vi "test Correct Acyclic Labels In Log.vi"(8 "error in":errorcluster, 11 "TestCase in":refnum<class "Logging Loopback.lvclass">) -> (0 "error out":errorcluster, 3 "TestCase out":refnum<class "Logging Loopback.lvclass">)   [LabVIEW 2020, in "Logging Loopback.lvclass"]
uses:
  Logging Loopback.lvclass
  C:/Users/nitest/Desktop/Git 2020/niveristand-custom-device-testing-tools/VeriStandTestCase/VeriStandTestCase.lvclass
  Logging Loopback.lvclass/Logging Loopback.ctl
  4890de3c-2bf7-434e-869c-ee5afaf04248.vi
  <vilib>/NI VeriStand/Execution/Workspace/NI VeriStand - Set Multiple Channel Values.vi
  <vilib>/WebDAVClient/Advanced/Get Buffer.vi
  <vilib>/addons/_JKI Toolkits/VI Tester/TestCase.llb/TestCase.lvclass
  <vilib>/WebDAVClient/NI_WebDAV.lvlib
  <vilib>/NI VeriStand/Execution/Workspace/NI_VS Workspace ExecutionAPI.lvlib
  C:/Program Files (x86)/National Instruments/LabVIEW 2020/vi.lib/addons/_JKI Toolkits/VI Tester/TestCase.llb/TestCase.lvclass
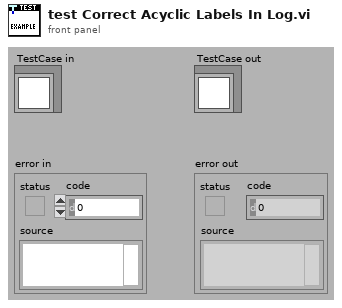
[diagram p1: front panel]
types:
  T1 = typedef "NI_WebDAV.lvlib/SessionHandle.ctl" = refnum<k1>
  T2 = typedef "NI_VS Workspace ExecutionAPI.lvlib/WorkspaceAPI.ctl" = refnum<k24>
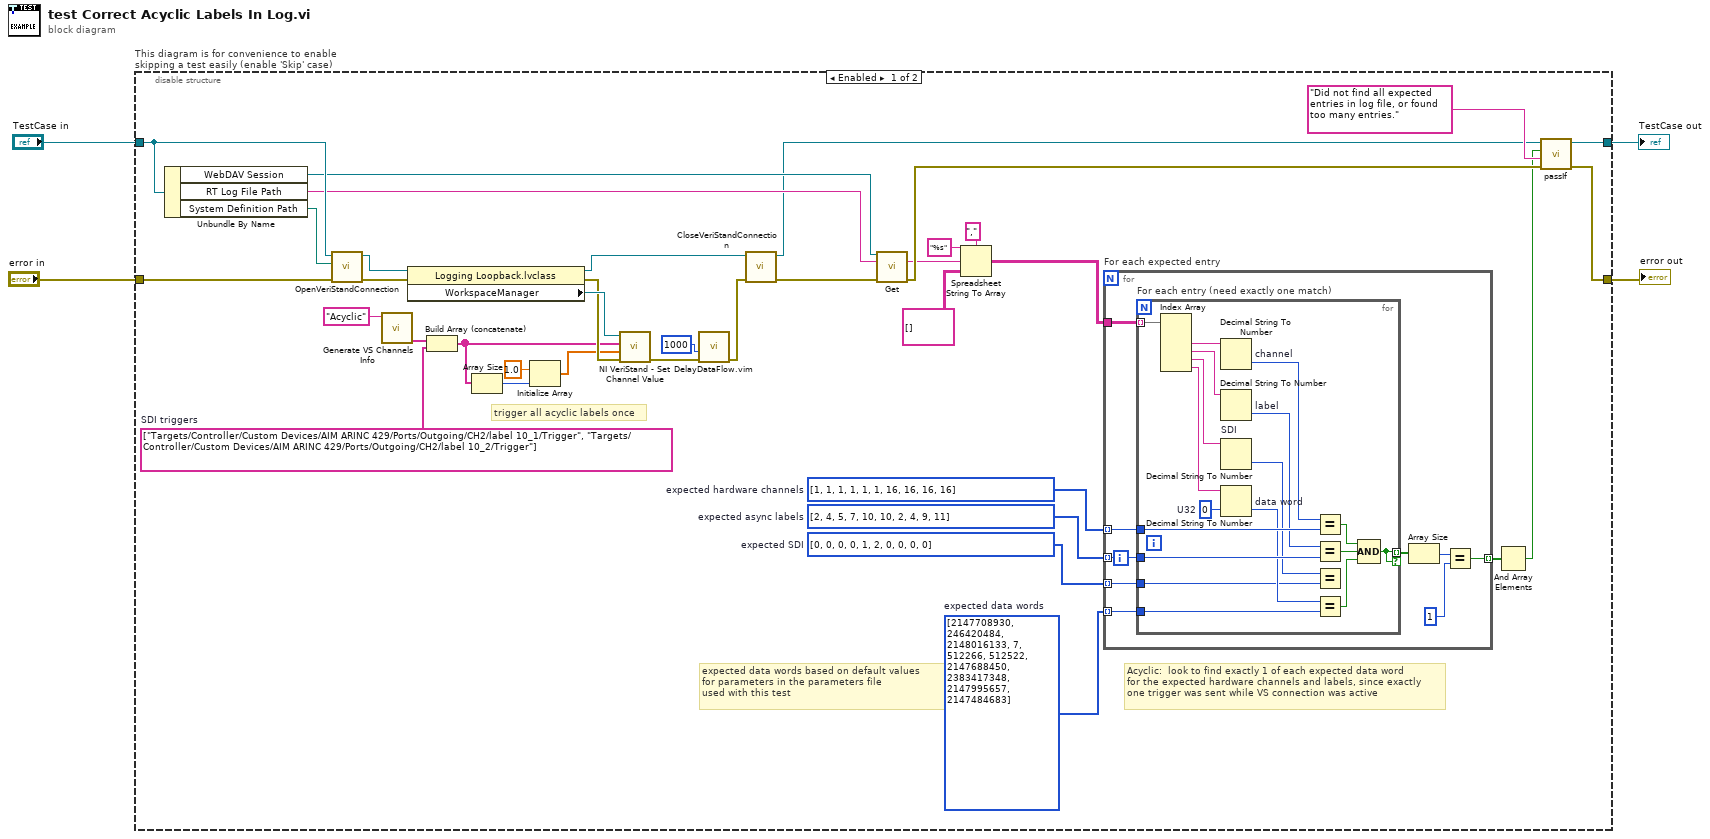
[diagram p0: block diagram]
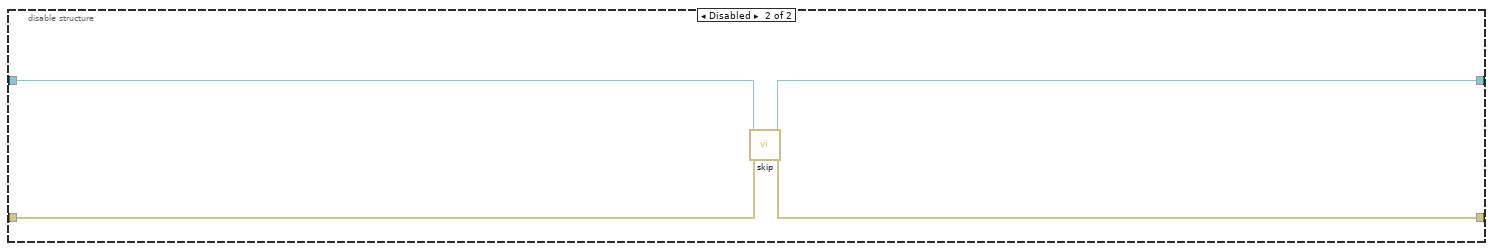
[diagram p2: hidden frame]
diagram:
  n1 = disable-structure "This diagram is for convenience to enable skipping a test easily (enable 'Skip' case)" shown="Enabled" {
    disable-tunnel: "TestCase in" -> [w39 w72]
    disable-tunnel: [w29 w70] -> w1
    disable-tunnel: [w30 w71] -> w3
    disable-tunnel: "error in" -> [w41 w69]
    frame Enabled {
      w6 = string[] ["Targets/Controller/Custom Devices/AIM ARINC 429/Ports/Outgoing/CH2/label 10_1/Trigger", "Targets/Controller/Custom Devices/AIM ARINC 429/Ports/Outgoing/CH2/label 10_2/Trigger"]  # SDI triggers
      w8 = i32[] [0, 0, 0, 0, 1, 2, 0, 0, 0, 0]  # expected SDI
      w23 = u32[] [2147708930, 246420484, 2148016133, 7, 512266, 512522, 2147688450, 2383417348, 2147995657, 2147484683]  # expected data words
      w25 = i32[] [1, 1, 1, 1, 1, 1, 16, 16, 16, 16]  # expected hardware channels
      w24 = i32[] [2, 4, 5, 7, 10, 10, 2, 4, 9, 11]  # expected async labels
      # "Acyclic:  look to find exactly 1 of each expected data word\nfor the expected hardware channels and labels, since exactly\none trigger was sent while VS connection was active"
      # "expected data words based on default values\nfor parameters in the parameters file\nused with this test"
      # "trigger all acyclic labels once"
      n2 = Unbundle By Name(w39) -> ("WebDAV Session"=w36:T1, "RT Log File Path"=w35:string, "System Definition Path"=w40:path)
      n3 = call-dynamic "OpenVeriStandConnection.vi"("error in (no error)"=w41, "System Definition File"=w40, "VeriStand Test Case in"=w39) -> ("error out"=w19:errorcluster, "VeriStand Test Case out"=w20:refnum<class "Logging Loopback.lvclass">)  [unwired: 6 in, 1 out]
      n4 = call "Generate VS Channels Info.vi"("Transfer Type"="Acyclic") -> ("Tx Trigger Channels Array"=w7:string[])  [unwired: 6 in, 4 out]
      n5 = property class="Logging Loopback.lvclass"(reference=w20, error in=w19) -> (reference out=w16:refnum<class "Logging Loopback.lvclass">, error out=w17:errorcluster, "WorkspaceManager"=w18:T2)
      n6 = Build Array (concatenate)(w7, w6) -> (w5:string[])
      n7 = Array Size(array=w5) -> (size(s)=w10:i32)
      n8 = Initialize Array(1.0, w10) -> (w12:dbl[])
      n9 = call-poly <vilib>:"NI VeriStand - Set Channel Value.vi"("error in (no error)"=w17, "Values"=w12, "Channels"=w5, "WorkspaceManager in"=w18) -> ("error out"=w14:errorcluster)  [unwired: 6 in, 1 out]
      n10 = call "DelayDataFlow.vim"("value in"=w14, "milliseconds to wait"=u32 1000) -> ("value out"=w13:errorcluster)  [unwired: 2 in, 1 out]
      n11 = call-dynamic "CloseVeriStandConnection.vi"("error in (no error)"=w13, "VeriStand Test Case in"=w16) -> ("error out"=w38:errorcluster, "VeriStand Test Case out"=w27:refnum<class "Logging Loopback.lvclass">)  [unwired: 8 in]
      n12 = call-poly <vilib>:"Get.vi"("session handle"=w36, "relative uri"=w35, "error in (no error)"=w38) -> ("data"=w34:string, "error out"=w37:errorcluster)  [unwired: 10 in, 1 out]
      n13 = Spreadsheet String To Array(delimiter (Tab)=",", format string="%s", spreadsheet string=w34, array type (2D Dbl)=string[][] []) -> (array=w26:string[][])
      n14 = for "For each expected entry" {
        tunnel: w25 -> [w49] mode=indexing
        tunnel: w24 -> [w48] mode=indexing
        tunnel: w23 -> [w47] mode=indexing
        tunnel: w26 -> [w50]
        tunnel: [w44] -> w22 mode=indexing
        tunnel: w8 -> [w42] mode=indexing
        n15 = for "For each entry (need exactly one match)" {
          tunnel: w50 -> [w68] mode=indexing
          tunnel: w49 -> [w63]
          tunnel: w48 -> [w64]
          tunnel: w47 -> [w65]
          tunnel: [w61] -> w45 mode=indexing if=w61
          tunnel: w42 -> [w53]
          w60 = u32 0  # U32
          n16 = Index Array(array=w68) -> (element #2=w67:string, element #3=w66:string, element #4=w52:string, element #5=w54:string)  [unwired: 5 in, 1 out]
          n17 = Decimal String To Number "channel"(string=w67) -> (number=w57:i32)  [unwired: 2 in, 1 out]
          n18 = Decimal String To Number "label"(string=w66) -> (number=w56:i32)  [unwired: 2 in, 1 out]
          n19 = Decimal String To Number "SDI"(string=w52) -> (number=w51:i32)  [unwired: 2 in, 1 out]
          n20 = Decimal String To Number "data word"(string=w54, default (0L)=w60) -> (number=w55:u32)  [unwired: 1 in, 1 out]
          n21 = Equal?(x=w57, y=w63) -> (x = y?=w59:bool)
          n22 = Equal?(x=w56, y=w64) -> (x = y?=w58:bool)
          n23 = Equal?(x=w51, y=w53) -> ()  [unwired: 1 out]
          n24 = Equal?(x=w55, y=w65) -> (x = y?=w62:bool)
          n25 = Compound Arithmetic op=AND(w59, w58, w62) -> (w61:bool)
        }
        n26 = Array Size(array=w45) -> (size(s)=w43:i32)
        n27 = Equal?(x=w43, y=1) -> (x = y?=w44:bool)
      }
      n28 = And Array Elements(Boolean array=w22) -> (logical AND=w21:bool)
      n29 = call-dynamic "passIf.vi"("error in (no error)"=w37, "message (\"\")"="Did not find all expected entries in log file, or found too many entries." ("message (\"\")"), "pass"=w21, "TestCase in"=w27) -> ("error out"=w30:errorcluster, "TestCase out"=w29:refnum<class "Logging Loopback.lvclass">)  [unwired: 6 in]
    }
    frame Disabled {
      # "skip test result while test is under development"
      n30 = call <vilib>:"skip.vi"("error in (no error)"=w69, "TestCase in"=w72) -> ("error out"=w71:errorcluster, "TestCase out"=w70:refnum<class "Logging Loopback.lvclass">)  [unwired: 8 in]
    }
  }
  "error out" <- w3
  "TestCase out" <- w1
